vi "PathBuild_Force.vi"(3 "Name_Test":string(combo)="D_L_", 4 "Lane_Number":string(combo)="ST1_", 5 "Date":string) -> (2 "path":path)   [LabVIEW 2017]
uses:
  <vilib>/Utility/file.llb/Write Delimited Spreadsheet (string).vi
panel:
  out "file or folder exists?":bool
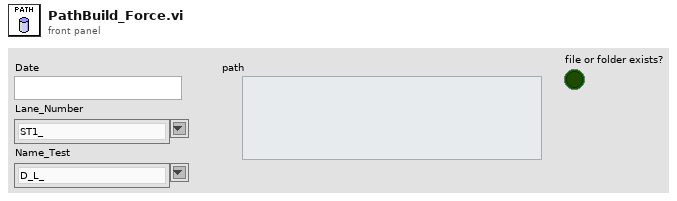
[diagram p1: front panel]
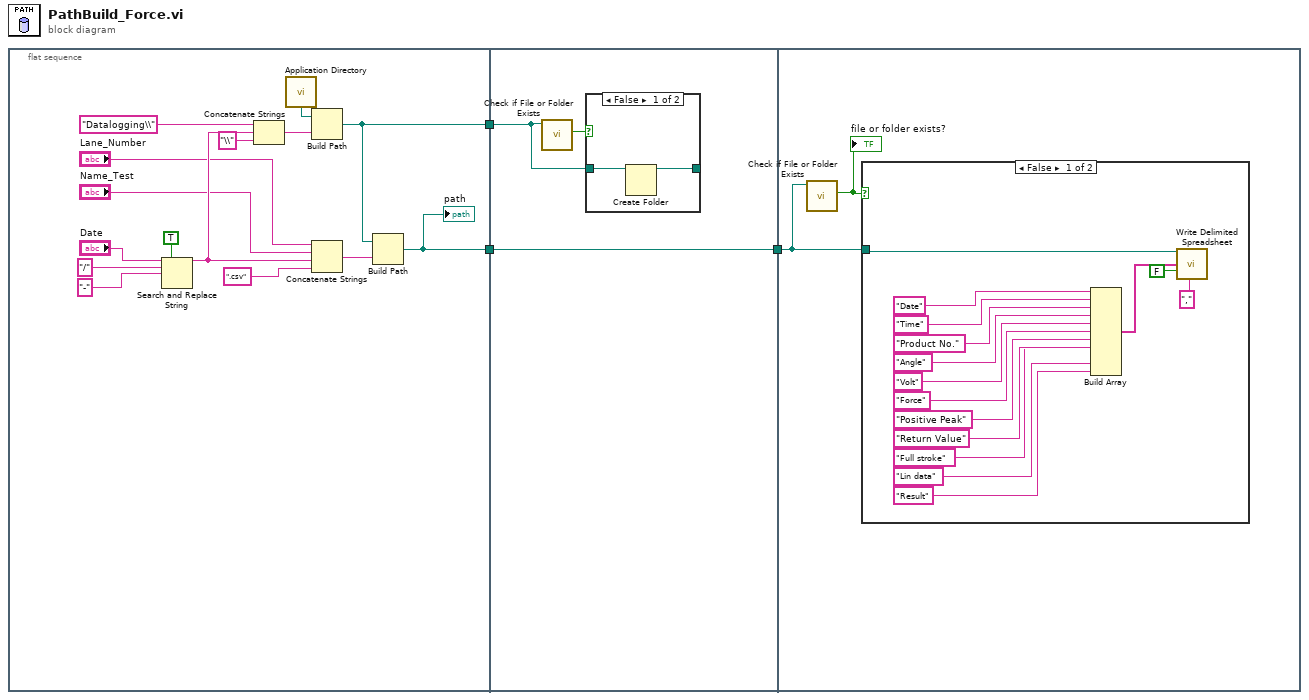
[diagram p0: block diagram]
diagram:
  n1 = flat-sequence {
    tunnel: [w7] -> w3
    tunnel: [w6] -> w1
    tunnel: w3 -> [w20]
    tunnel: [w19] -> w2
    tunnel: w1 -> [w19]
    tunnel: w2 -> [w25]
    frame #0 {
      n2 = Search and Replace String(replace all?=TRUE ("replace all? (F)"), input string="Date", search string="/" ("input string"), replace string="-" ("replace string (\"\")")) -> (result string=w11:string)  [unwired: 4 in, 3 out]
      n3 = Concatenate Strings("Datalogging\\", w11, "\\" ("string")) -> (w8:string)
      n4 = call <vilib>:"Application Directory.vi"() -> ("Application Directory"=w9:path)
      n5 = Build Path(base path=w9, name or relative path=w8) -> (appended path=w7:path)
      n6 = Concatenate Strings("Lane_Number", "Name_Test", w11, ".csv" ("string")) -> (w13:string)
      n7 = Build Path(base path=w7, name or relative path=w13) -> (appended path=w6:path)
      "path" <- w6
    }
    frame #1 {
      n8 = call <vilib>:"Check if File or Folder Exists.vi"("path"=w20) -> ("file or folder exists?"=w21:bool)  [unwired: 8 in, 2 out]
      n9 = case shown="False" w21 {
        tunnel: w20 -> [w23 w24]
        tunnel: [w22 w24] -> _
        frame False {
          n10 = Create Folder(path (use dialog)=w23) -> (created path=w22:path)  [unwired: 2 in, 2 out]
        }
        frame True {
        }
      }
    }
    frame #2 {
      n11 = call <vilib>:"Check if File or Folder Exists.vi"("path"=w25) -> ("file or folder exists?"=w26:bool)  [unwired: 8 in, 2 out]
      "file or folder exists?" <- w26
      n12 = case shown="False" w26 {
        tunnel: w25 -> [w33 _]
        frame False {
          n13 = Build Array("Date", "Time", "Product No.", "Angle", "Volt", "Force", "Positive Peak", "Return Value", "Full stroke", "Lin data", "Result") -> (w36:string[])
          n14 = call-poly <vilib>:"Write Delimited Spreadsheet.vi"("file path (dialog if empty)"=w33, "1D data"=w36, "append to file? (new file:F)"=FALSE, "delimiter (\\t)"="," ("delimiter (\\t)")) -> ()  [unwired: 10 in, 2 out]
        }
        frame True {
        }
      }
    }
  }
